vi "PIDAdjustment.vi"(0 "StopPIDAdjEvn":refnum<user-event>, 4 "ref PID Set Value":refnum<vi>, 5 "TestType":enum16{"Normal", "Stall"}(ring), 6 "DynoValue_PID":refnum<vi>, 7 "Close Loop Graph":refnum<vi>, 8 "ManTaskQ":refnum<queue>, 9 "FuncBtn":refnum<vi>[](array[refnum]), 10 "Conditions":refnum<vi>[](array[refnum]), 11 "PIDValue":refnum<vi>[](array[refnum])) -> ()   [LabVIEW 2024]
uses:
  MFActor/MainFormTaskName.ctl
  PIDAdjProcStep.ctl
panel:
  out "YScalMax":dbl
  out "LeavePIDAdj":refnum<vi>
  in  "PID Set Value":dbl
  out "CloseLoopHiValue":bool
  in  "DelayDwell(ms)":u32
  out "Close Loop Value Lo":refnum<vi>
  out "Close Loop Value Hi":refnum<vi>
  out "Close Loop Value Dwell":refnum<vi>
  out "Close Loop Value Speed":refnum<vi>
  out "DirnPID":refnum<vi>
  in  "DirnPID":enum16{"CW", "CCW"}(ring) caption="轉向"
  in  "Close Loop Value Speed":i32 caption="轉速(RPM)"
  in  "Close Loop Value Dwell":dbl caption="時間(s)"
  in  "Close Loop Value Lo":dbl caption="扭力低值(N.m)"
  in  "Close Loop Value Hi":dbl caption="扭力高值(N.m)"
  out "NDS":refnum<vi>
  out "NIS":refnum<vi>
  out "ND":refnum<vi>
  out "NI":refnum<vi>
  out "NPS":refnum<vi>
  out "NP":refnum<vi>
  in  "NDS":enum16{"A", "B", "C", "D", "E", "F", "G", "H"}(ring)
  in  "ND":dbl(slide) caption="D" scale=0.0..99.0 scale format="%.3f"
  in  "NIS":enum16{"A", "B", "C", "D", "E", "F", "G", "H"}(ring)
  in  "NI":dbl(slide) caption="I" scale=0.0..99.0 scale format="%.3f"
  in  "NPS":enum16{"A", "B", "C", "D", "E", "F", "G", "H"}(ring)
  in  "NP":dbl(slide) caption="P" scale=0.0..99.0 scale format="%.3f"
  out "ClearCloseLoopGraph":refnum<vi>
  out "PID Adj.End":refnum<vi>
  out "PID Adj.Start":refnum<vi>
  in  "ClearCloseLoopGraph":bool
  in  "PID Adj.End":bool
  in  "PID Adj.Start":bool
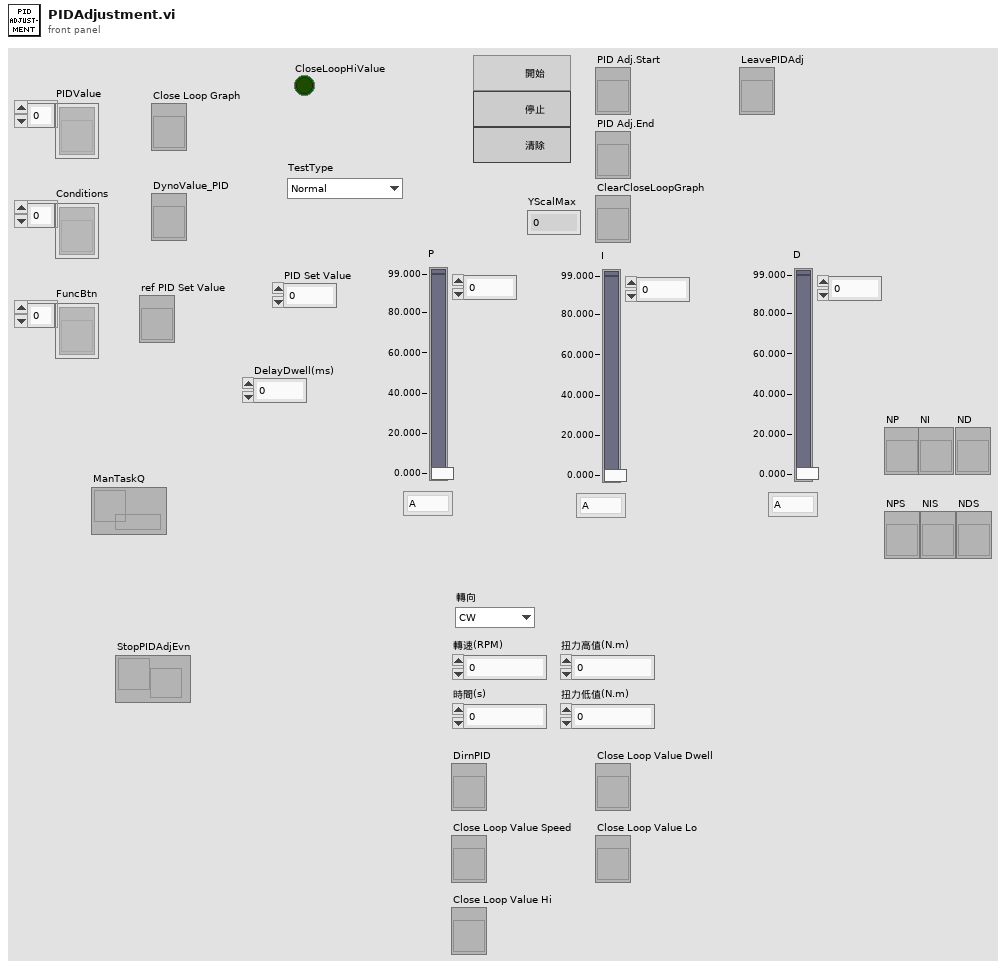
[diagram p1: front panel]
types:
  T1 = typedef "PIDAdjProcStep.ctl" = enum16{"None", "Delay(ms)", "Init", "ZeroSpeed", "StopRunPID", "RunPID", "PlotCurve", "HighLowChange", "End"}
  T2 = typedef "MainFormTaskName.ctl" = enum16{"None", "InitMainForUI", "InitInterfaceCards", "OpenDIOCard", "CloseDIOCard", "OpenAIOCard", "CloseAIOCard", "OpenRED", "CloseRED", "Open4503B", "Close4503B", "OpenPW3390", "ClosePW3390", "Open4118", "Close4118", "OpenPID", "ClosePID", "OpenRmtService", "CloseRmtService", "QueryData", "ZeroAngle", "ErrCodeHandler", "RestError", "DIHandler", "SendDO", "SendAO", "LoadRecipe", "RefreshPIDUI", "WriteRecipe", "EditMultiPt", "LoadSetting", "WriteSetting", "InitDev", "CloseDev", "SetDriverTQ", "SetTorque", "DriveSinTQ", "SinTorque", "SetSpeed", "ActiveMotor", "RunPID", "StartRunPIDAdj", "InitAutoUI", "RefreshAutoUI", "LeaveAutoTestUI", "UpdateRecipeContent", "StartTestProc", "StopTestProc", "CleanTestData", "InitCalibration", "LeaveCalibration", "Calibration", "SelectExportedFileType", "ExportAsCSV", "ExportAsXls", "SoftwareReady", "ShowPSMsg", "DCPowerCtrl", "AllProcClosed", "ExitApp"}
  T3 = cluster{"PIDAdjProcStep":T1, "millisecond timer value":u32}
  T4 = cluster{"Speed":dbl, "Troque":dbl, "Watts":dbl, "Angle":dbl}
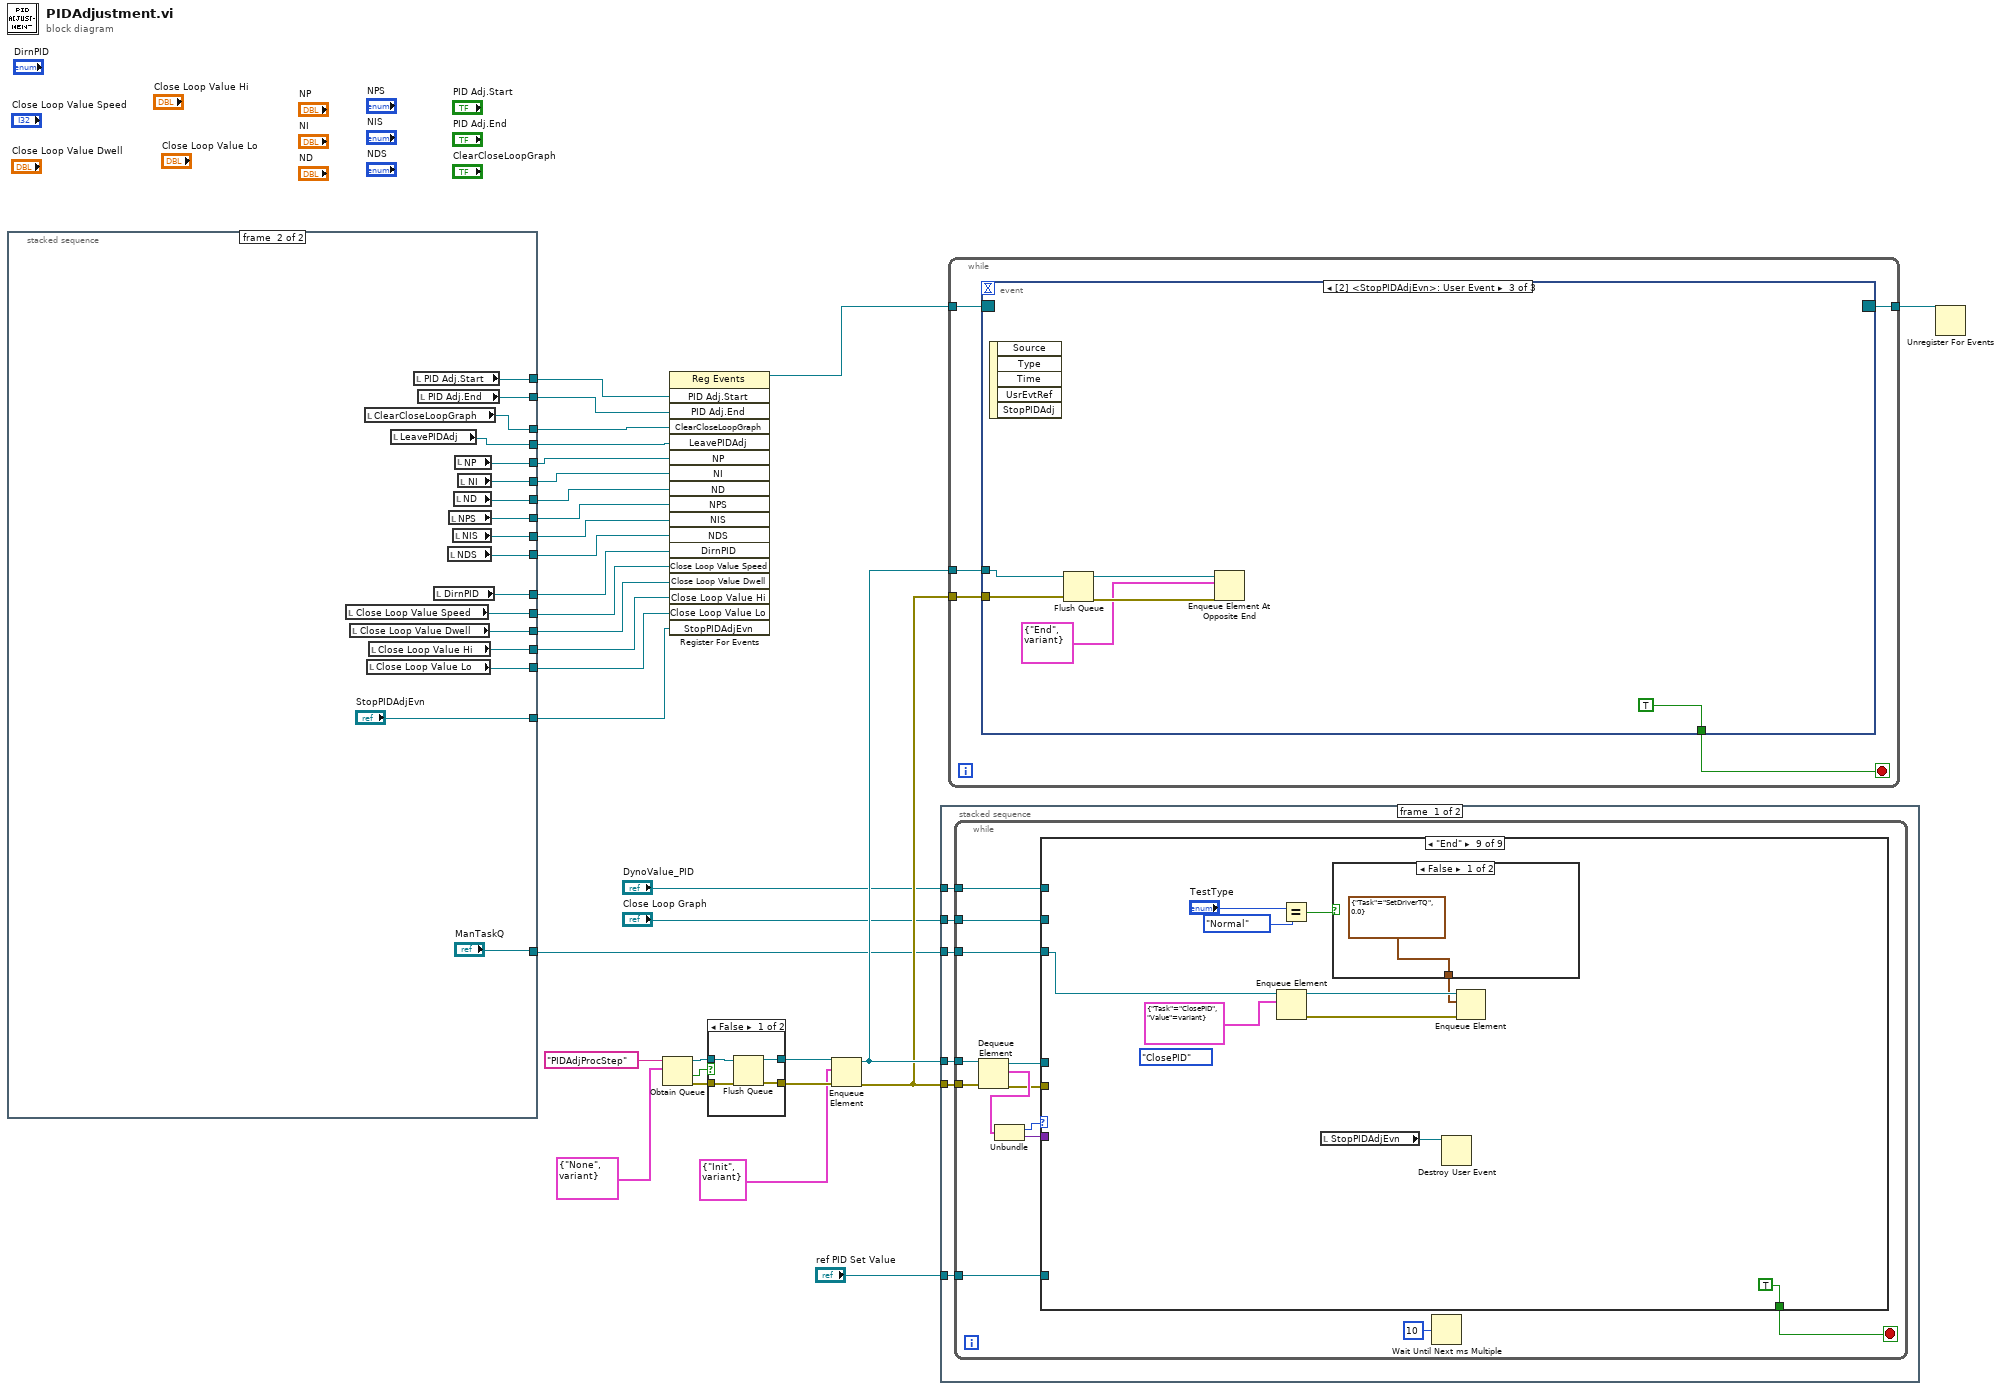
[diagram p0: block diagram]
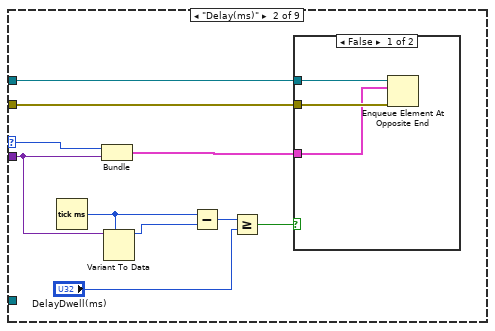
[diagram p3: hidden frame]
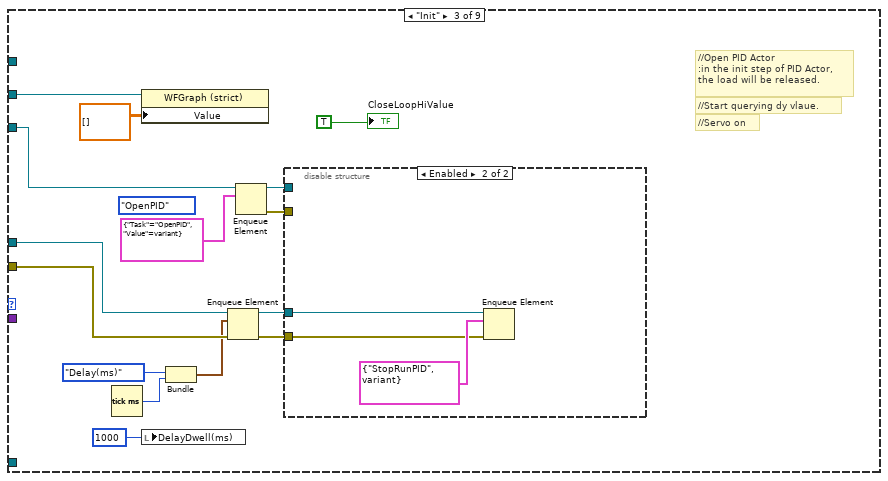
[diagram p5: hidden frame]
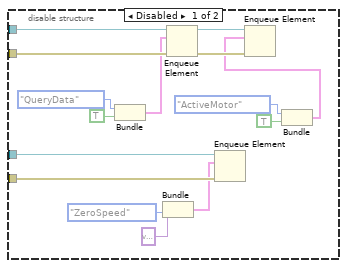
[diagram p6: hidden frame]
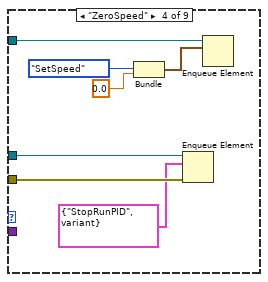
[diagram p7: hidden frame]
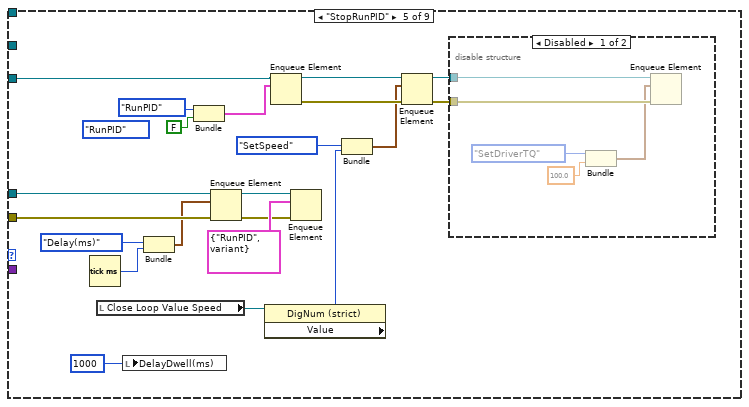
[diagram p8: hidden frame]
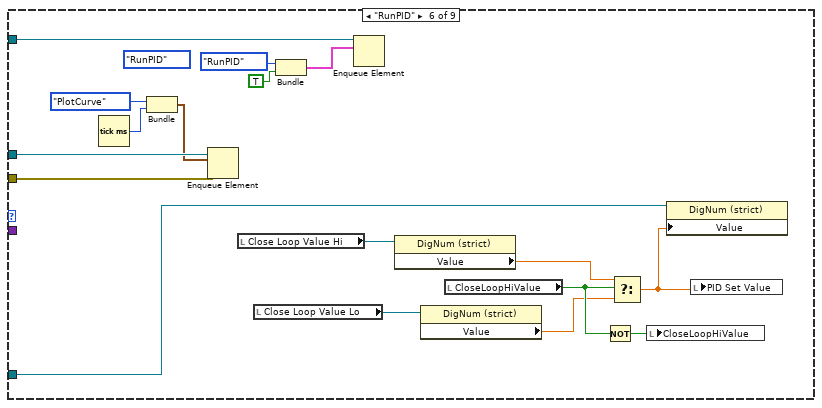
[diagram p10: hidden frame]
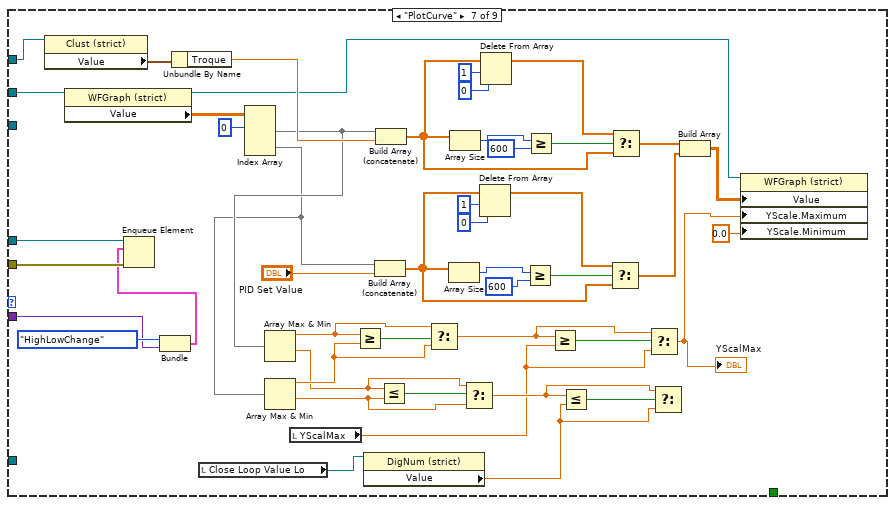
[diagram p11: hidden frame]
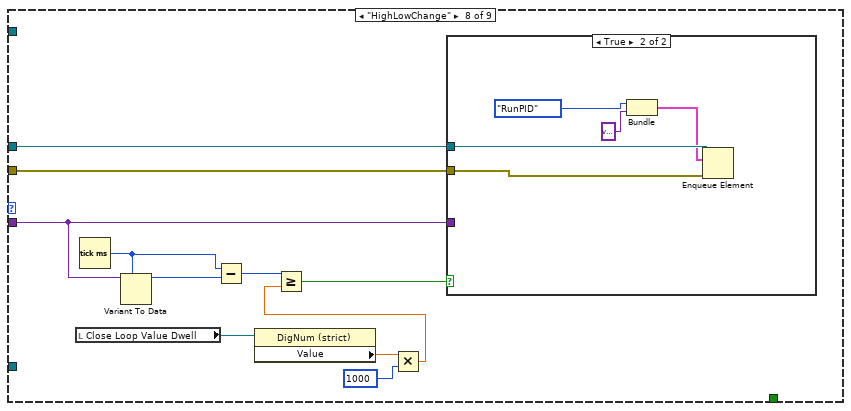
[diagram p12: hidden frame]
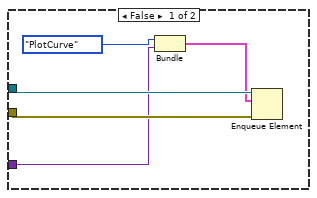
[diagram p13: hidden frame]
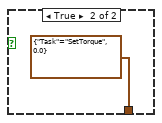
[diagram p14: hidden frame]
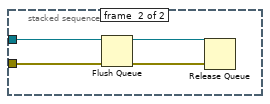
[diagram p15: hidden frame]
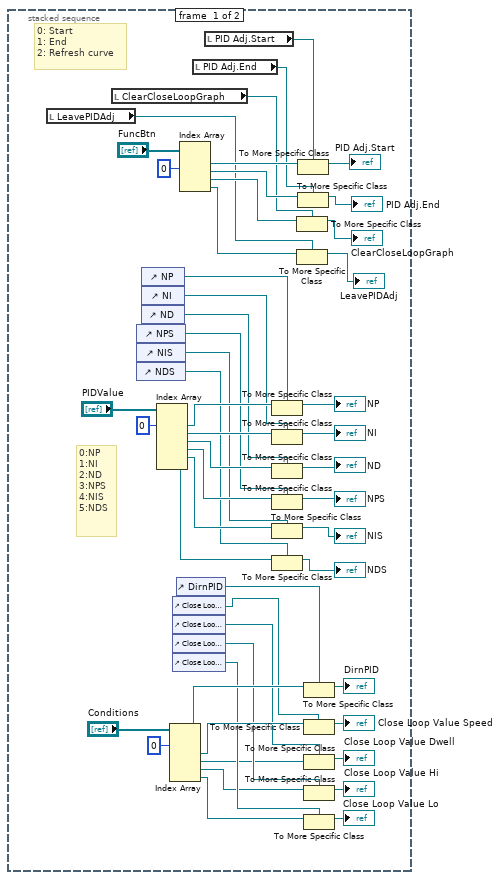
[diagram p17: hidden frame]
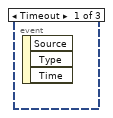
[diagram p18: hidden frame]
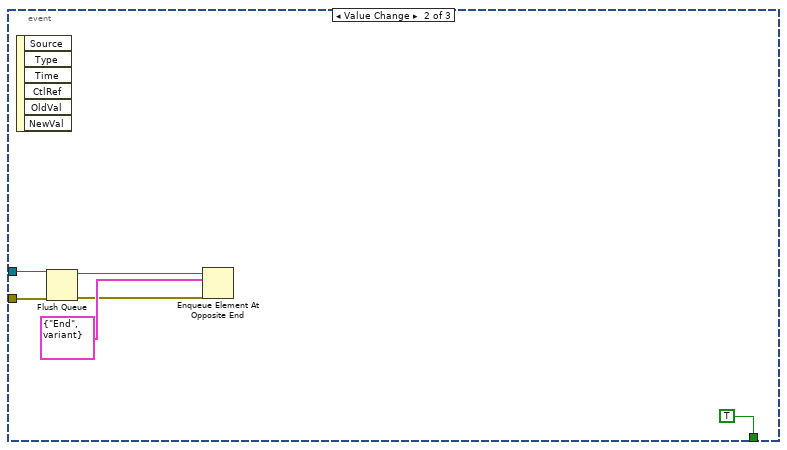
[diagram p19: hidden frame]
diagram:
  n1 = stacked-sequence {
    tunnel: [_ w100] -> w31
    tunnel: [_ w99] -> w30
    tunnel: [_ w98] -> w29
    tunnel: [_ w97] -> w28
    tunnel: [_ w96] -> w27
    tunnel: [_ w95] -> w26
    tunnel: [_ w94] -> w25
    tunnel: [_ w93] -> w24
    tunnel: [_ w92] -> w23
    tunnel: [_ w91] -> w22
    tunnel: [_ w90] -> w21
    tunnel: [_ w89] -> w20
    tunnel: [_ w88] -> w19
    tunnel: [_ w87] -> w18
    tunnel: [_ w86] -> w3
    tunnel: [_ "StopPIDAdjEvn"] -> w2
    tunnel: [_ "ManTaskQ"] -> w1
    frame #0 {
      # "0:NP\n1:NI\n2:ND\n3:NPS\n4:NIS\n5:NDS"
      # "0: Start\n1: End\n2: Refresh curve"
      n2 = local read "LeavePIDAdj"() -> (w34:refnum<vi>)
      n3 = local read "ClearCloseLoopGraph"() -> (w75:refnum<vi>)
      n4 = control-ref of="NPS"() -> (w61:refnum<vi>)
      n5 = control-ref of="NIS"() -> (w60:refnum<vi>)
      n6 = control-ref of="NDS"() -> (w59:refnum<vi>)
      n7 = control-ref of="NP"() -> (w64:refnum<vi>)
      n8 = control-ref of="NI"() -> (w63:refnum<vi>)
      n9 = control-ref of="ND"() -> (w62:refnum<vi>)
      n10 = Index Array(array="PIDValue", index #1=0 ("index")) -> (element #1=w70:refnum<vi>, element #2=w69:refnum<vi>, element #3=w68:refnum<vi>, element #4=w67:refnum<vi>, element #5=w66:refnum<vi>, element #6=w65:refnum<vi>)  [unwired: 5 in]
      n11 = Index Array(array="Conditions", index #1=0 ("index")) -> (element #1=w50:refnum<vi>, element #2=w49:refnum<vi>, element #3=w38:refnum<vi>, element #4=w37:refnum<vi>, element #5=w36:refnum<vi>)  [unwired: 4 in]
      n12 = control-ref of="Close Loop Value Speed"() -> (w47:refnum<vi>)
      n13 = control-ref of="Close Loop Value Dwell"() -> (w46:refnum<vi>)
      n14 = control-ref of="Close Loop Value Hi"() -> (w45:refnum<vi>)
      n15 = control-ref of="Close Loop Value Lo"() -> (w44:refnum<vi>)
      n16 = control-ref of="DirnPID"() -> (w48:refnum<vi>)
      n17 = Index Array(array="FuncBtn", index #1=0 ("index")) -> (element #1=w81:refnum<vi>, element #2=w80:refnum<vi>, element #3=w79:refnum<vi>, element #4=w35:refnum<vi>)  [unwired: 3 in]
      n18 = local read "PID Adj.End"() -> (w76:refnum<vi>)
      n19 = local read "PID Adj.Start"() -> (w78:refnum<vi>)
      n20 = To More Specific Class(target class=w64, reference=w70) -> (specific class reference=→"NP":refnum<vi>)  [unwired: 1 in, 1 out]
      n21 = To More Specific Class(target class=w63, reference=w69) -> (specific class reference=→"NI":refnum<vi>)  [unwired: 1 in, 1 out]
      n22 = To More Specific Class(target class=w62, reference=w68) -> (specific class reference=→"ND":refnum<vi>)  [unwired: 1 in, 1 out]
      n23 = To More Specific Class(target class=w61, reference=w67) -> (specific class reference=→"NPS":refnum<vi>)  [unwired: 1 in, 1 out]
      n24 = To More Specific Class(target class=w60, reference=w66) -> (specific class reference=→"NIS":refnum<vi>)  [unwired: 1 in, 1 out]
      n25 = To More Specific Class(target class=w59, reference=w65) -> (specific class reference=→"NDS":refnum<vi>)  [unwired: 1 in, 1 out]
      n26 = To More Specific Class(target class=w75, reference=w79) -> (specific class reference=→"ClearCloseLoopGraph":refnum<vi>)  [unwired: 1 in, 1 out]
      n27 = To More Specific Class(target class=w34, reference=w35) -> (specific class reference=→"LeavePIDAdj":refnum<vi>)  [unwired: 1 in, 1 out]
      n28 = To More Specific Class(target class=w78, reference=w81) -> (specific class reference=→"PID Adj.Start":refnum<vi>)  [unwired: 1 in, 1 out]
      n29 = To More Specific Class(target class=w76, reference=w80) -> (specific class reference=→"PID Adj.End":refnum<vi>)  [unwired: 1 in, 1 out]
      n30 = To More Specific Class(target class=w48, reference=w50) -> (specific class reference=→"DirnPID":refnum<vi>)  [unwired: 1 in, 1 out]
      n31 = To More Specific Class(target class=w47, reference=w49) -> (specific class reference=→"Close Loop Value Speed":refnum<vi>)  [unwired: 1 in, 1 out]
      n32 = To More Specific Class(target class=w46, reference=w38) -> (specific class reference=→"Close Loop Value Dwell":refnum<vi>)  [unwired: 1 in, 1 out]
      n33 = To More Specific Class(target class=w45, reference=w37) -> (specific class reference=→"Close Loop Value Hi":refnum<vi>)  [unwired: 1 in, 1 out]
      n34 = To More Specific Class(target class=w44, reference=w36) -> (specific class reference=→"Close Loop Value Lo":refnum<vi>)  [unwired: 1 in, 1 out]
    }
    frame #1 {
      n35 = local read "Close Loop Value Speed"() -> (w90:refnum<vi>)
      n36 = local read "Close Loop Value Dwell"() -> (w89:refnum<vi>)
      n37 = local read "ClearCloseLoopGraph"() -> (w98:refnum<vi>)
      n38 = local read "Close Loop Value Lo"() -> (w87:refnum<vi>)
      n39 = local read "Close Loop Value Hi"() -> (w88:refnum<vi>)
      n40 = local read "LeavePIDAdj"() -> (w86:refnum<vi>)
      n41 = local read "PID Adj.Start"() -> (w100:refnum<vi>)
      n42 = local read "PID Adj.End"() -> (w99:refnum<vi>)
      n43 = local read "DirnPID"() -> (w91:refnum<vi>)
      n44 = local read "NDS"() -> (w92:refnum<vi>)
      n45 = local read "NPS"() -> (w94:refnum<vi>)
      n46 = local read "NIS"() -> (w93:refnum<vi>)
      n47 = local read "ND"() -> (w95:refnum<vi>)
      n48 = local read "NP"() -> (w97:refnum<vi>)
      n49 = local read "NI"() -> (w96:refnum<vi>)
    }
  }
  n50 = Obtain Queue(name (unnamed)="PIDAdjProcStep", element data type=cluster{"PIDAdjProcStep":T1, variant} {"PIDAdjProcStep"=enum."None", variant}) -> (queue out=w14:refnum<queue>, created new?=w12:bool, error out=w13:errorcluster)  [unwired: 3 in]
  n51 = register-events(w31, w30, w29, w3, w28, w27, w26, w25, w24, w23, w22, w21, w20, w19, w18, w2) -> (reference out=w32:refnum<event-registration>)  [unwired: 2 in, 1 out]
  n52 = case shown="False" w12 {
    tunnel: w14 -> [w104 w106]
    tunnel: w13 -> [w103 w105]
    tunnel: [w102 w106] -> w11
    tunnel: [w101 w105] -> w10
    frame False {
      n53 = Flush Queue(queue=w104, error in (no error)=w103) -> (queue out=w102:refnum<queue>, error out=w101:errorcluster)  [unwired: 1 out]
    }
    frame True {
    }
  }
  n54 = Enqueue Element(queue=w11, element=cluster{"PIDAdjProcStep":T1, variant} {"PIDAdjProcStep"=enum."Init", variant}, error in (no error)=w10) -> (queue out=w8:refnum<queue>, error out=w7:errorcluster)  [unwired: 1 in, 1 out]
  n55 = stacked-sequence {
    tunnel: w8 -> [w112 w305]
    tunnel: w7 -> [w111 w304]
    tunnel: "DynoValue_PID" -> [w110 _]
    tunnel: "Close Loop Graph" -> [w109 _]
    tunnel: w1 -> [w108 _]
    tunnel: "ref PID Set Value" -> [w107 _]
    frame #0 {
      n56 = while {
        tunnel: w112 -> [w125]
        tunnel: w111 -> [w124]
        tunnel: w110 -> [w114]
        tunnel: w109 -> [w117]
        tunnel: w108 -> [w116]
        tunnel: w107 -> [w113]
        stop <- w118 stop-if-true
        n57 = Dequeue Element(queue=w125, error in (no error)=w124) -> (queue out=w120:refnum<queue>, element=w123:cluster{"PIDAdjProcStep":T1, variant}, error out=w119:errorcluster)  [unwired: 1 in, 1 out]
        n58 = Unbundle(w123) -> ("PIDAdjProcStep"=w122:T1, w121:variant)
        n59 = case shown="\"End\"" w122 {
          selector: w122 -> [_ w128 _ _ _ _ _ _ _]
          tunnel: w121 -> [_ w127 _ _ _ _ w229 w271 _]
          tunnel: w120 -> [_ w130 w150 w174 w186 w221 w233 w270 _]
          tunnel: w119 -> [_ w129 w149 w173 w185 w220 w232 w269 _]
          tunnel: [_ _ _ _ _ _ _ _ TRUE] -> w118
          tunnel: w117 -> [_ _ w153 _ _ _ w268 _ _]
          tunnel: w116 -> [_ _ w142 w178 w198 w208 _ _ w297]
          tunnel: w114 -> [_ _ _ _ _ _ w265 _ _]
          tunnel: w113 -> [_ _ _ _ _ w210 _ _ _]
          frame "None", Default {
          }
          frame "Delay(ms)" {
            n60 = Tick Count (ms)() -> (millisecond timer value=w135:u32)
            n61 = Bundle("PIDAdjProcStep"=w128, w127) -> (w126:cluster{"PIDAdjProcStep":T1, variant})  [unwired: 1 in]
            n62 = Variant To Data(type=w135, Variant=w127) -> (data=w134:u32)  [unwired: 1 in, 1 out]
            n63 = Subtract(x=w135, y=w134) -> (x-y=w133:u32)
            n64 = Greater Or Equal?(x=w133, y="DelayDwell(ms)") -> (x >= y?=w131:bool)
            n65 = case shown="False" w131 {
              tunnel: w130 -> [w138 _]
              tunnel: w129 -> [w137 _]
              tunnel: w126 -> [w136 _]
              frame False {
                n66 = Enqueue Element At Opposite End(queue=w138, element=w136, error in (no error)=w137) -> ()  [unwired: 1 in, 3 out]
              }
              frame True {
              }
            }
          }
          frame "Init" {
            (unwired) MainFormTaskName."OpenPID" ("Task")
            # "//Servo on"
            # "//Start querying dy vlaue."
            # "//Open PID Actor\n:in the init step of PID Actor,\nthe load will be released."
            n67 = Tick Count (ms)() -> (millisecond timer value=w147:u32)
            n68 = property class="WFGraph (strict)"(reference=w153, "Value"=dbl[][] []) -> ()  [unwired: 1 in, 2 out]
            n69 = local write "DelayDwell(ms)"(u32 1000) -> ()
            n70 = Bundle("PIDAdjProcStep"=PIDAdjProcStep."Delay(ms)", "millisecond timer value"=w147) -> (w146:T3)  [unwired: 1 in]
            n71 = Enqueue Element(queue=w150, element=w146, error in (no error)=w149) -> (queue out=w145:refnum<queue>, error out=w144:errorcluster)  [unwired: 1 in, 1 out]
            n72 = Enqueue Element(queue=w142, element=cluster{"Task":T2, "Value":variant} {"Task"=enum."OpenPID", "Value"=variant}) -> (queue out=w140:refnum<queue>, error out=w139:errorcluster)  [unwired: 2 in, 1 out]
            n73 = disable-structure shown="Enabled" {
              disable-tunnel: w145 -> [w168 w170]
              disable-tunnel: w144 -> [w167 w169]
              disable-tunnel: w140 -> [w163 _]
              disable-tunnel: w139 -> [w162 _]
              frame Disabled {
                n74 = Bundle("Task"=MainFormTaskName."QueryData", TRUE) -> (w159:cluster{"Task":T2, bool})  [unwired: 1 in]
                n75 = Bundle("PIDAdjProcStep"=PIDAdjProcStep."ZeroSpeed", variant) -> (w164:cluster{"PIDAdjProcStep":T1, variant})  [unwired: 1 in]
                n76 = Enqueue Element(queue=w163, element=w159, error in (no error)=w162) -> (queue out=w158:refnum<queue>, error out=w157:errorcluster)  [unwired: 1 in, 1 out]
                n77 = Enqueue Element(queue=w168, element=w164, error in (no error)=w167) -> ()  [unwired: 1 in, 3 out]
                n78 = Bundle("Task"=MainFormTaskName."ActiveMotor", TRUE) -> (w154:cluster{"Task":T2, bool})  [unwired: 1 in]
                n79 = Enqueue Element(queue=w158, element=w154, error in (no error)=w157) -> ()  [unwired: 1 in, 3 out]
              }
              frame Enabled {
                n80 = Enqueue Element(queue=w170, element=cluster{"PIDAdjProcStep":T1, variant} {"PIDAdjProcStep"=enum."StopRunPID", variant}, error in (no error)=w169) -> ()  [unwired: 1 in, 3 out]
              }
            }
            "CloseLoopHiValue" <- TRUE
          }
          frame "ZeroSpeed" {
            n81 = Bundle("Task"=MainFormTaskName."SetSpeed", 0.0) -> (w175:cluster{"Task":T2, dbl})  [unwired: 1 in]
            n82 = Enqueue Element(queue=w174, element=cluster{"PIDAdjProcStep":T1, variant} {"PIDAdjProcStep"=enum."StopRunPID", variant}, error in (no error)=w173) -> ()  [unwired: 1 in, 3 out]
            n83 = Enqueue Element(queue=w178, element=w175) -> ()  [unwired: 2 in, 3 out]
          }
          frame "StopRunPID" {
            (unwired) MainFormTaskName."RunPID" ("Task")
            n84 = Tick Count (ms)() -> (millisecond timer value=w181:u32)
            n85 = local read "Close Loop Value Speed"() -> (w191:refnum<vi>)
            n86 = local write "DelayDwell(ms)"(u32 1000) -> ()
            n87 = Bundle("PIDAdjProcStep"=PIDAdjProcStep."Delay(ms)", "millisecond timer value"=w181) -> (w179:T3)  [unwired: 1 in]
            n88 = Bundle("Task"=MainFormTaskName."RunPID", FALSE) -> (w195:cluster{"Task":T2, bool})  [unwired: 1 in]
            n89 = Enqueue Element(queue=w186, element=w179, error in (no error)=w185) -> (queue out=w184:refnum<queue>, error out=w183:errorcluster)  [unwired: 1 in, 1 out]
            n90 = property class="DigNum (strict)"(reference=w191) -> ("Value"=w190:i32)  [unwired: 1 in, 2 out]
            n91 = Enqueue Element(queue=w198, element=w195) -> (queue out=w194:refnum<queue>, error out=w193:errorcluster)  [unwired: 2 in, 1 out]
            n92 = Enqueue Element(queue=w184, element=cluster{"PIDAdjProcStep":T1, variant} {"PIDAdjProcStep"=enum."RunPID", variant}, error in (no error)=w183) -> ()  [unwired: 1 in, 3 out]
            n93 = Bundle("Task"=MainFormTaskName."SetSpeed", "Value"=w190) -> (w189:cluster{"Task":T2, "Value":i32})  [unwired: 1 in]
            n94 = Enqueue Element(queue=w194, element=w189, error in (no error)=w193) -> (queue out=w188:refnum<queue>, error out=w187:errorcluster)  [unwired: 1 in, 1 out]
            n95 = disable-structure shown="Disabled" {
              disable-tunnel: w188 -> [w204 _]
              disable-tunnel: w187 -> [w203 _]
              frame Disabled {
                n96 = Bundle("Task"=MainFormTaskName."SetDriverTQ", 100.0) -> (w200:cluster{"Task":T2, dbl})  [unwired: 1 in]
                n97 = Enqueue Element(queue=w204, element=w200, error in (no error)=w203) -> ()  [unwired: 1 in, 3 out]
              }
              frame Enabled {
              }
            }
          }
          frame "RunPID" {
            (unwired) MainFormTaskName."RunPID" ("Task")
            n98 = Tick Count (ms)() -> (millisecond timer value=w218:u32)
            n99 = Bundle("PIDAdjProcStep"=PIDAdjProcStep."PlotCurve", "millisecond timer value"=w218) -> (w217:T3)  [unwired: 1 in]
            n100 = Enqueue Element(queue=w221, element=w217, error in (no error)=w220) -> ()  [unwired: 1 in, 3 out]
            n101 = local read "Close Loop Value Hi"() -> (w214:refnum<vi>)
            n102 = local read "Close Loop Value Lo"() -> (w212:refnum<vi>)
            n103 = Bundle("Task"=MainFormTaskName."RunPID", TRUE) -> (w205:cluster{"Task":T2, bool})  [unwired: 1 in]
            n104 = Enqueue Element(queue=w208, element=w205) -> ()  [unwired: 2 in, 3 out]
            n105 = property class="DigNum (strict)"(reference=w214) -> ("Value"=w213:dbl)  [unwired: 1 in, 2 out]
            n106 = property class="DigNum (strict)"(reference=w212) -> ("Value"=w211:dbl)  [unwired: 1 in, 2 out]
            n107 = local read "CloseLoopHiValue"() -> (w216:bool)
            n108 = Not(x=w216) -> (.not. x?=w215:bool)
            n109 = Select(t=w213, s=w216, f=w211) -> (s? t:f=w209:dbl)
            n110 = local write "CloseLoopHiValue"(w215) -> ()
            n111 = property class="DigNum (strict)"(reference=w210, "Value"=w209) -> ()  [unwired: 1 in, 2 out]
            n112 = local write "PID Set Value"(w209) -> ()
          }
          frame "PlotCurve" {
            n113 = property class="Clust (strict)"(reference=w265) -> ("Value"=w264:T4)  [unwired: 1 in, 2 out]
            n114 = property class="WFGraph (strict)"(reference=w268) -> (reference out=w245:refnum<vi>, "Value"=w267:dbl[][])  [unwired: 1 in, 1 out]
            n115 = Bundle("PIDAdjProcStep"=PIDAdjProcStep."HighLowChange", w229) -> (w230:cluster{"PIDAdjProcStep":T1, variant})  [unwired: 1 in]
            n116 = Enqueue Element(queue=w233, element=w230, error in (no error)=w232) -> ()  [unwired: 1 in, 3 out]
            n117 = Unbundle By Name(w264) -> ("Troque"=w263:dbl)
            n118 = local read "Close Loop Value Lo"() -> (w237:refnum<vi>)
            n119 = Index Array(array=w267, index (row) #1=0 ("index (row)")) -> (element #1=w243:dbl[], element #2=w242:dbl[])  [unwired: 3 in]
            n120 = Array Max & Min(array=w243) -> (max value=w228:dbl, min value=w227:dbl)  [unwired: 2 out]
            n121 = Array Max & Min(array=w242) -> (max value=w240:dbl, min value=w238:dbl)  [unwired: 2 out]
            n122 = local read "YScalMax"() -> (w223:dbl)
            n123 = Greater Or Equal?(x=w228, y=w240) -> (x >= y?=w241:bool)
            n124 = property class="DigNum (strict)"(reference=w237) -> ("Value"=w234:dbl)  [unwired: 1 in, 2 out]
            n125 = Build Array (concatenate)(w242, "PID Set Value") -> (w255:dbl[])
            n126 = Build Array (concatenate)(w243, w263) -> (w256:dbl[])
            n127 = Less Or Equal?(x=w227, y=w238) -> (x <= y?=w239:bool)
            n128 = Select(t=w228, s=w241, f=w240) -> (s? t:f=w226:dbl)
            n129 = Array Size(array=w255) -> (size(s)=w251:i32)
            n130 = Array Size(array=w256) -> (size(s)=w260:i32)
            n131 = Select(t=w227, s=w239, f=w238) -> (s? t:f=w225:dbl)
            n132 = Delete From Array(array=w255, length=1, index=0) -> (array with subset deleted=w254:dbl[])  [unwired: 1 out]
            n133 = Delete From Array(array=w256, length=1, index=0) -> (array with subset deleted=w257:dbl[])  [unwired: 1 out]
            n134 = Greater Or Equal?(x=w251, y=600) -> (x >= y?=w250:bool)
            n135 = Greater Or Equal?(x=w260, y=600) -> (x >= y?=w261:bool)
            n136 = Greater Or Equal?(x=w226, y=w223) -> (x >= y?=w236:bool)
            n137 = Less Or Equal?(x=w225, y=w234) -> (x <= y?=w235:bool)
            n138 = Select(t=w254, s=w250, f=w255) -> (s? t:f=w246:dbl[])
            n139 = Select(t=w257, s=w261, f=w256) -> (s? t:f=w247:dbl[])
            n140 = Select(t=w226, s=w236, f=w223) -> (s? t:f=w222:dbl)
            "YScalMax" <- w222
            n141 = Select(t=w225, s=w235, f=w234) -> ()  [unwired: 1 out]
            n142 = Build Array(w247, w246) -> (w244:dbl[][])
            n143 = property class="WFGraph (strict)"(reference=w245, "Value"=w244, "YScale.Maximum"=w222, "YScale.Minimum"=0.0 ("Y Scale.Range:Minimum")) -> ()  [unwired: 1 in, 2 out]
          }
          frame "HighLowChange" {
            n144 = local read "Close Loop Value Dwell"() -> (w276:refnum<vi>)
            n145 = Tick Count (ms)() -> (millisecond timer value=w279:u32)
            n146 = Variant To Data(type=w279, Variant=w271) -> (data=w278:u32)  [unwired: 1 in, 1 out]
            n147 = Subtract(x=w279, y=w278) -> (x-y=w277:u32)
            n148 = property class="DigNum (strict)"(reference=w276) -> ("Value"=w275:dbl)  [unwired: 1 in, 2 out]
            n149 = Multiply(x=w275, y=1000) -> (x*y=w273:dbl)
            n150 = Greater Or Equal?(x=w277, y=w273) -> (x >= y?=w272:bool)
            n151 = case shown="True" w272 {
              tunnel: w271 -> [w280 _]
              tunnel: w270 -> [w284 w289]
              tunnel: w269 -> [w283 w288]
              frame False {
                n152 = Bundle("PIDAdjProcStep"=PIDAdjProcStep."PlotCurve", w280) -> (w281:cluster{"PIDAdjProcStep":T1, variant})  [unwired: 1 in]
                n153 = Enqueue Element(queue=w284, element=w281, error in (no error)=w283) -> ()  [unwired: 1 in, 3 out]
              }
              frame True {
                n154 = Bundle("PIDAdjProcStep"=PIDAdjProcStep."RunPID", variant) -> (w285:cluster{"PIDAdjProcStep":T1, variant})  [unwired: 1 in]
                n155 = Enqueue Element(queue=w289, element=w285, error in (no error)=w288) -> ()  [unwired: 1 in, 3 out]
              }
            }
          }
          frame "End" {
            (unwired) MainFormTaskName."ClosePID" ("Task")
            n156 = Enqueue Element(queue=w297, element=cluster{"Task":T2, "Value":variant} {"Task"=enum."ClosePID", "Value"=variant}) -> (queue out=w294:refnum<queue>, error out=w293:errorcluster)  [unwired: 2 in, 1 out]
            n157 = Equal?(x="TestType", y=enum16{"Normal", "Stall"}."Normal") -> (x = y?=w292:bool)
            n158 = local read "StopPIDAdjEvn"() -> (w290:refnum<user-event>)
            n159 = case shown="False" w292 {
              tunnel: [cluster{"Task":T2, dbl} {"Task"=enum."SetDriverTQ", 0.0} ("element") cluster{"Task":T2, dbl} {"Task"=enum."SetTorque", 0.0} ("element")] -> w291
              frame False {
              }
              frame True {
              }
            }
            n160 = Destroy User Event(user event=w290) -> ()  [unwired: 1 in, 1 out]
            n161 = Enqueue Element(queue=w294, element=w291, error in (no error)=w293) -> ()  [unwired: 1 in, 3 out]
          }
        }
        n162 = Wait Until Next ms Multiple(millisecond multiple=u32 10) -> ()  [unwired: 1 out]
      }
    }
    frame #1 {
      n163 = Flush Queue(queue=w305, error in (no error)=w304) -> (queue out=w303:refnum<queue>, error out=w302:errorcluster)  [unwired: 1 out]
      n164 = Release Queue(queue=w303, error in (no error)=w302) -> ()  [unwired: 1 in, 3 out]
    }
  }
  n165 = while {
    tunnel: w32 -> [w310]
    tunnel: [w308] -> w17
    tunnel: w8 -> [w307]
    tunnel: w7 -> [w306]
    stop <- w309 stop-if-true
    n166 = event shown="[2] <StopPIDAdjEvn>: User Event" {
      selector: w310 -> [_ _ _]
      dyn-events: [_ _ _] -> w308
      timeout: _ -> [_ _ _]
      tunnel: [_ TRUE TRUE] -> w309
      tunnel: w307 -> [_ w314 w320]
      tunnel: w306 -> [_ w313 w319]
      event Timeout {
        n167 = event-data() -> ()  [unwired: 1 in, 3 out]
      }
      event Value Change {
        n168 = event-data() -> ()  [unwired: 1 in, 6 out]
        n169 = Flush Queue(queue=w314, error in (no error)=w313) -> (queue out=w312:refnum<queue>, error out=w311:errorcluster)  [unwired: 1 out]
        n170 = Enqueue Element At Opposite End(queue=w312, element=cluster{"PIDAdjProcStep":T1, variant} {"PIDAdjProcStep"=enum."End", variant}, error in (no error)=w311) -> ()  [unwired: 1 in, 3 out]
      }
      event User Event {
        n171 = event-data() -> ()  [unwired: 1 in, 5 out]
        n172 = Flush Queue(queue=w320, error in (no error)=w319) -> (queue out=w322:refnum<queue>, error out=w321:errorcluster)  [unwired: 1 out]
        n173 = Enqueue Element At Opposite End(queue=w322, element=cluster{"PIDAdjProcStep":T1, variant} {"PIDAdjProcStep"=enum."End", variant}, error in (no error)=w321) -> ()  [unwired: 1 in, 3 out]
      }
    }
  }
  n174 = Unregister For Events(event registration refnum=w17) -> ()  [unwired: 1 in, 1 out]
